vi "settings_to_cluster_singleVI.vi"(1 "Version":string, 2 "vi reference 2":refnum<vi>) -> (3 "error out":errorcluster, 4 "VI Name":string, 5 "XML String":string, 6 "vi reference":refnum<vi>)   [LabVIEW 2019]
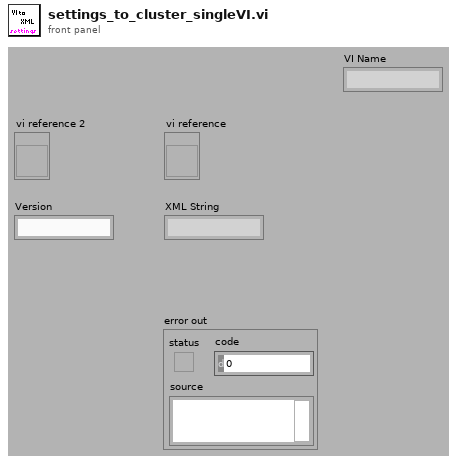
[diagram p1: front panel]
types:
  T1 = cluster{"Name":string, "Version":string, "Controls":cluster{"Name":string, "Data":string}[]}
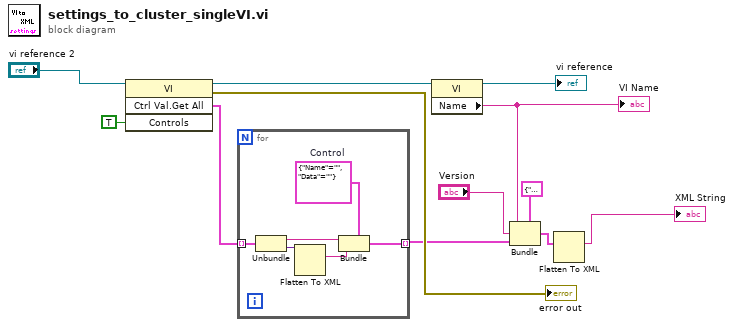
[diagram p0: block diagram]
diagram:
  n1 = invoke class="VI" method="Ctrl Val.Get All"(reference="vi reference 2", "Controls"=TRUE) -> (reference out=w9:refnum<vi>, error out=→"error out":errorcluster, "Get All Control Values Variant"=w12:cluster{"Name":string, "Variant Data":variant}[])  [unwired: 2 in, 1 out]
  n2 = for {
    tunnel: w12 -> [w15] mode=indexing
    tunnel: [w14] -> w4 mode=indexing
    w13 = cluster{"Name":string, "Data":string} {"Name"="", "Data"=""}  # Control
    n3 = Unbundle(w15) -> ("Name"=w16:string, "Variant Data"=w17:variant)
    n4 = Flatten To XML(anything=w17) -> (xml string=w18:string)
    n5 = Bundle(cluster=w13, "Name"=w16, "Data"=w18) -> (w14:cluster{"Name":string, "Data":string})
  }
  n6 = property class="VI"(reference=w9) -> (reference out=→"vi reference":refnum<vi>, "Name"=w2:string)  [unwired: 1 in, 1 out]
  "VI Name" <- w2
  n7 = Bundle(cluster=T1 {"Name"="", "Version"="", "Controls"=[]}, "Name"=w2, "Version"="Version", "Controls"=w4) -> (w5:T1)
  n8 = Flatten To XML(anything=w5) -> (xml string=→"XML String":string)
